vi "Generate Sync Pulse.vi"(0 "generate sync pulse (strobe)":bool, 2 "resources":T1={"sync pulse resources"={"sync pulse destination terminal"="", "sync100"="", "sync pulse source terminal"="", "imported sync pulse register"="", "generate sync pulse handshake"="", "enable sync pulse register"="", "sync pulse clock"=""}, "serial channel resources"={"sc 0"={"completed frames register"=""}, "sc 1"={"completed frames register"=""}, "sc 2"={"completed frames register"=""}, "sc 3"={"completed frames register"=""}, "sc 4"={"completed frames register"=""}, "sc 5"={"completed frames register"=""}, "sc 6"={"completed frames register"=""}, "sc 7"={"completed frames register"=""}}, "dram manager 0"={"DRAM class"=refnum, "process clock"="", "registers"={"configuration"={"write time slice"="", "request time slice"="", "DRAM arbiter config"="", "partition config"=""}, "reset"={"handshake"={"start.go"="", "start.go rcvd"="", "done.go"="", "done.go rcvd"=""}, "process"={"in"="", "out"=""}, "write"={"in"="", "out 0"="", "out 1"="", "out 2"="", "out 3"=""}, "read"={"in"="", "out 0"="", "out 1"="", "out 2"="", "out 3"=""}}, "status"={"partition full"=""}}, "FIFOs"={"write data"={"FIFO 0"="", "FIFO 1"="", "FIFO 2"="", "FIFO 3"=""}, "request metadata"={"FIFO"=""}, "read data VOQ"={"FIFO 0"="", "FIFO 1"="", "FIFO 2"="", "FIFO 3"=""}, "read data"={"FIFO 0"="", "FIFO 1"="", "FIFO 2"="", "FIFO 3"=""}}, "num active streams"=0.0, "max open read requests"=256}, "dram manager 1"={"DRAM class"=refnum, "process clock"="", "registers"={"configuration"={"write time slice"="", "request time slice"="", "DRAM arbiter config"="", "partition config"=""}, "reset"={"handshake"={"start.go"="", "start.go rcvd"="", "done.go"="", "done.go rcvd"=""}, "process"={"in"="", "out"=""}, "write"={"in"="", "out 0"="", "out 1"="", "out 2"="", "out 3"=""}, "read"={"in"="", "out 0"="", "out 1"="", "out 2"="", "out 3"=""}}, "status"={"partition full"=""}}, "FIFOs"={"write data"={"FIFO 0"="", "FIFO 1"="", "FIFO 2"="", "FIFO 3"=""}, "request metadata"={"FIFO"=""}, "read data VOQ"={"FIFO 0"="", "FIFO 1"="", "FIFO 2"="", "FIFO 3"=""}, "read data"={"FIFO 0"="", "FIFO 1"="", "FIFO 2"="", "FIFO 3"=""}}, "num active streams"=0.0, "max open read requests"=256}}, 5 "enable sync pulse":bool) -> (4 "sync pulse out":bool)   [LabVIEW 2020, in "GettingStarted_Common_148X_FPGA.lvlib"]
uses:
  GettingStarted_Common_148X_FPGA.lvlib
  Types/Common Resources.ctl
  <instrlib>/_niInstr/Memory/v1/FPGA/DRAM/niInstr Memory DRAM v1 FPGA.lvclass
  <instrlib>/FlexRIO/CSI-2/v2/FPGA/Types/Sync Pulse Resources.ctl
  Types/Serial Channel Resources.ctl
  Types/Single Serial Channel Resources.ctl
  <instrlib>/FlexRIO/CSI-2/v2/FPGA/DRAM Manager/Private/DRAM Manager.ctl
  <instrlib>/FlexRIO/CSI-2/v2/FPGA/DRAM Manager/Private/Common/DRAM Manager Registers.ctl
  <instrlib>/FlexRIO/CSI-2/v2/FPGA/DRAM Manager/Private/Common/Handshake Registers.ctl
  <instrlib>/FlexRIO/CSI-2/v2/FPGA/DRAM Manager/Private/Common/DRAM Manager FIFOs.ctl
  <instrlib>/FlexRIO/CSI-2/v2/FPGA/DRAM Manager/Private/Common/Write Data FIFO Ref.ctl
  <instrlib>/FlexRIO/CSI-2/v2/FPGA/DRAM Manager/Private/Common/Read Request Metadata FIFO Ref.ctl
  <instrlib>/FlexRIO/CSI-2/v2/FPGA/DRAM Manager/Private/Common/Read Data FIFO Ref.ctl
  <instrlib>/FlexRIO/CSI-2/v2/FPGA/NI CSI-2 API FPGA v2.lvlib
  <instrlib>/FlexRIO/CSI-2/v2/FPGA/DRAM Manager/DRAM Manager v2.lvlib
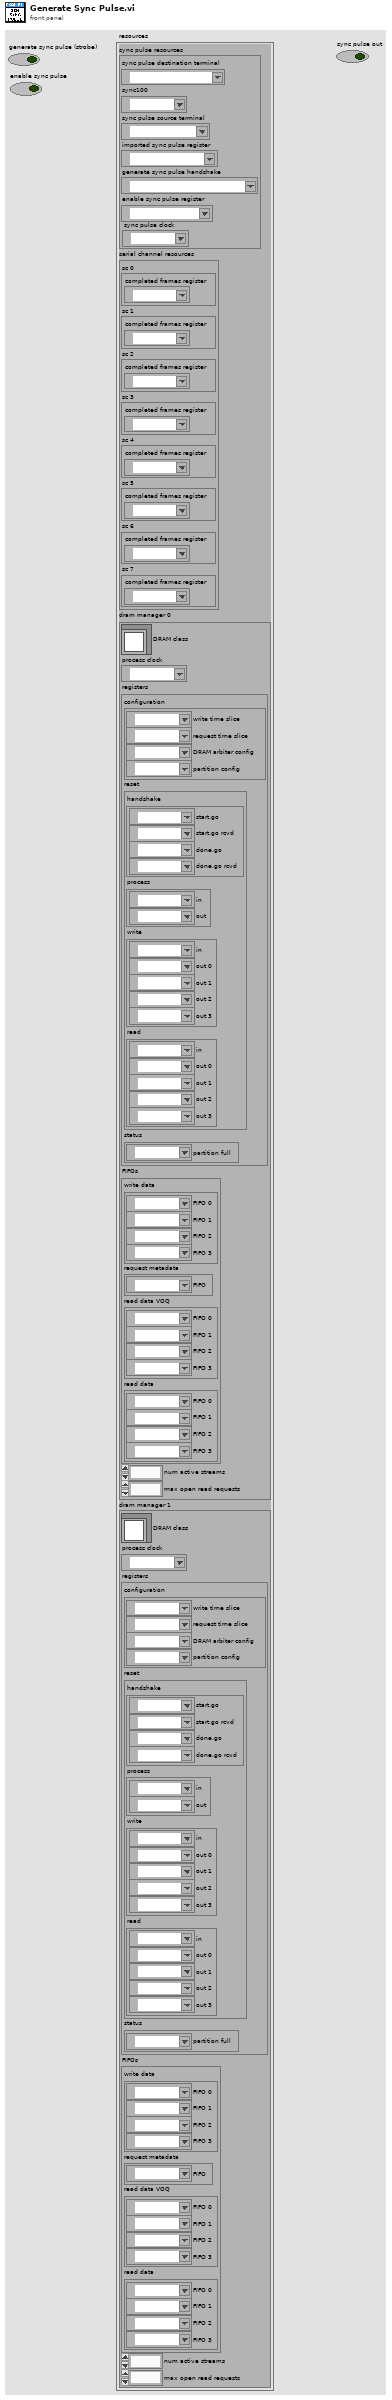
[diagram p1: front panel]
types:
  T1 = typedef "GettingStarted_Common_148X_FPGA.lvlib/Common Resources.ctl" = cluster{"sync pulse resources":T2, "serial channel resources":T3, "dram manager 0":T5, "dram manager 1":T5}
  T2 = typedef "NI CSI-2 API FPGA v2.lvlib/Sync Pulse Resources.ctl" = cluster{"sync pulse destination terminal":refnum<k21>, "sync100":refnum<k21>, "sync pulse source terminal":refnum<k21>, "imported sync pulse register":refnum<k21>, "generate sync pulse handshake":refnum<k21>, "enable sync pulse register":refnum<k21>, "sync pulse clock":refnum<k21>}
  T3 = typedef "GettingStarted_Common_148X_FPGA.lvlib/Serial Channel Resources.ctl" = cluster{"sc 0":T4, "sc 1":T4, "sc 2":T4, "sc 3":T4, "sc 4":T4, "sc 5":T4, "sc 6":T4, "sc 7":T4}
  T4 = typedef "GettingStarted_Common_148X_FPGA.lvlib/Single Serial Channel Resources.ctl" = cluster{"completed frames register":refnum<k21>}
  T5 = typedef "DRAM Manager v2.lvlib/DRAM Manager.ctl" = cluster{"DRAM class":refnum<class "niInstr Memory DRAM v1 FPGA.lvclass">, "process clock":refnum<k21>, "registers":T6, "FIFOs":T8, "num active streams":fxp<+,3,3>, "max open read requests":u16}
  T6 = typedef "DRAM Manager v2.lvlib/DRAM Manager Registers.ctl" = cluster{"configuration":cluster{"write time slice":refnum<k21>, "request time slice":refnum<k21>, "DRAM arbiter config":refnum<k21>, "partition config":refnum<k21>}, "reset":cluster{"handshake":T7, "process":cluster{"in":refnum<k21>, "out":refnum<k21>}, "write":cluster{"in":refnum<k21>, "out 0":refnum<k21>, "out 1":refnum<k21>, "out 2":refnum<k21>, "out 3":refnum<k21>}, "read":cluster{"in":refnum<k21>, "out 0":refnum<k21>, "out 1":refnum<k21>, "out 2":refnum<k21>, "out 3":refnum<k21>}}, "status":cluster{"partition full":refnum<k21>}}
  T7 = typedef "DRAM Manager v2.lvlib/Handshake Registers.ctl" = cluster{"start.go":refnum<k21>, "start.go rcvd":refnum<k21>, "done.go":refnum<k21>, "done.go rcvd":refnum<k21>}
  T8 = typedef "DRAM Manager v2.lvlib/DRAM Manager FIFOs.ctl" = cluster{"write data":cluster{"FIFO 0":T9, "FIFO 1":T9, "FIFO 2":T9, "FIFO 3":T9}, "request metadata":cluster{"FIFO":T10}, "read data VOQ":cluster{"FIFO 0":T11, "FIFO 1":T11, "FIFO 2":T11, "FIFO 3":T11}, "read data":cluster{"FIFO 0":T11, "FIFO 1":T11, "FIFO 2":T11, "FIFO 3":T11}}
  T9 = typedef "DRAM Manager v2.lvlib/Write Data FIFO Ref.ctl" = refnum<k21>
  T10 = typedef "DRAM Manager v2.lvlib/Read Request Metadata FIFO Ref.ctl" = refnum<k21>
  T11 = typedef "DRAM Manager v2.lvlib/Read Data FIFO Ref.ctl" = refnum<k21>
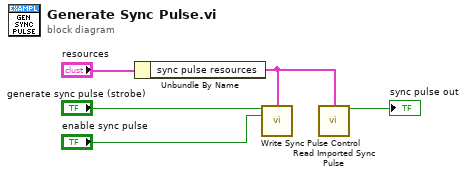
[diagram p0: block diagram]
diagram:
  n1 = Unbundle By Name("resources") -> ("sync pulse resources"=w5:T2)
  n2 = call <instrlib>:"Write Sync Pulse Control.vi"("generate sync pulse (strobe)"="generate sync pulse (strobe)", "sync pulse resources"=w5, "enable sync pulse"="enable sync pulse") -> ()  [unwired: 13 in]
  n3 = call <instrlib>:"Read Imported Sync Pulse.vi"("sync pulse resources"=w5) -> ("imported sync pulse"=→"sync pulse out":bool)  [unwired: 14 in]
